vi "Set Slide Range.vi"(9 "Max":i32, 10 "error in (no error)":errorcluster, 11 "Slide in":refnum<vi>) -> (2 "error out":errorcluster)   [LabVIEW 2021, in "GUI.lvlib"]
uses:
  GUI.lvlib
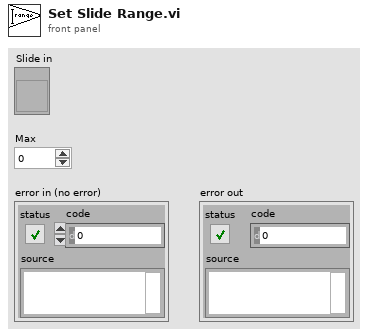
[diagram p1: front panel]
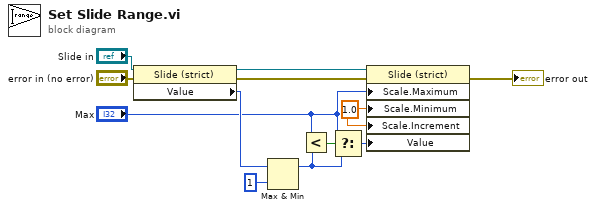
[diagram p0: block diagram]
diagram:
  w3 = 1.0 ("Scale.Range:Minimum")
  n1 = property class="Slide (strict)"(reference="Slide in", error in="error in (no error)") -> (reference out=w4:refnum<vi>, error out=w5:errorcluster, "Value"=w9:u16)
  n2 = Max & Min(x=w9, y=u16 1) -> (max(x,y)=w11:u16)  [unwired: 1 out]
  n3 = Less?(x="Max", y=w11) -> (x < y?=w6:bool)
  n4 = Select(t="Max", s=w6, f=w11) -> (s? t:f=w8:i32)
  n5 = property class="Slide (strict)"(reference=w4, error in=w5, "Scale.Maximum"="Max", "Scale.Minimum"=w3, "Scale.Increment"=w3, "Value"=w8) -> (error out=→"error out":errorcluster)  [unwired: 1 out]
